vi "Run_Post Core.vi"(0 "functionbase in":refnum<class "functionbase.lvclass">, 11 "error in (no error)":errorcluster) -> (4 "functionbase out":refnum<class "functionbase.lvclass">, 6 "Go to Run Pre Core?":bool, 15 "error out":errorcluster)   [LabVIEW 2019, in "LSL.lvlib" / "functionbase.lvclass"]
uses:
  functionbase.lvclass
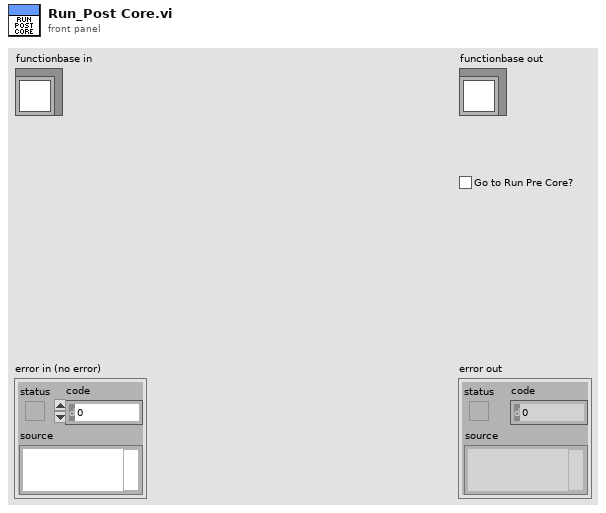
[diagram p1: front panel]
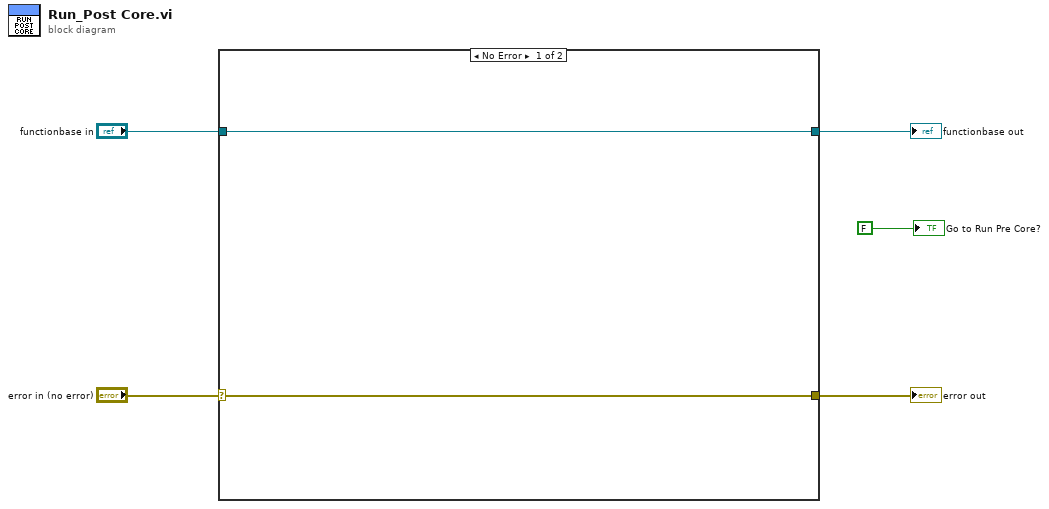
[diagram p0: block diagram]
diagram:
  n1 = case shown="No Error" "error in (no error)" {
    selector: "error in (no error)" -> [w6 w9]
    tunnel: [w6 w9] -> w4
    tunnel: [w7 w8] -> w2
    tunnel: "functionbase in" -> [w7 w8]
    frame No Error {
    }
    frame Error {
    }
  }
  "error out" <- w4
  "functionbase out" <- w2
  "Go to Run Pre Core?" <- FALSE ("Go to Run Pre Core?")
